vi "SpinnyCloseMotor.vi"(0 "Arduino Resource":T1={"VISA resource"="", "Board Type"=enum."Uno", "Connection Type"=enum."USB / Serial", "Bytes Per Packet (15)"=15}, 5 "error in":errorcluster) -> ()   [LabVIEW 2014]
uses:
  <vilib>/LabVIEW Interface for Arduino/Type Defs/Arduino Resource.ctl
  <vilib>/LabVIEW Interface for Arduino/Type Defs/Board Type.ctl
  <vilib>/LabVIEW Interface for Arduino/LabVIEW Interface for Arduino.lvlib
panel:
  in  "Stepper #":u8=1
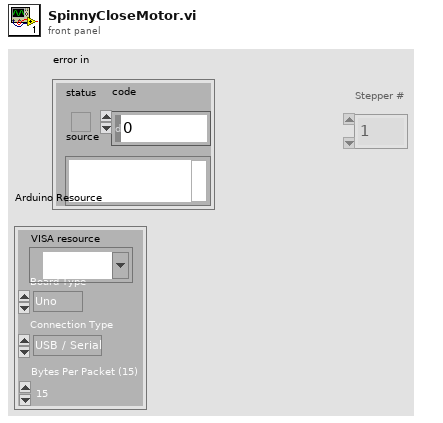
[diagram p1: front panel]
types:
  T1 = typedef "LabVIEW Interface for Arduino.lvlib/Arduino Resource.ctl" = cluster{"VISA resource":refnum<visa-resource-name>, "Board Type":T2, "Connection Type":enum8{"USB / Serial"}, "Bytes Per Packet (15)":u8}
  T2 = typedef "LabVIEW Interface for Arduino.lvlib/Board Type.ctl" = enum16{"Uno", "Dimuelanove w/Atmega 328", "Mega 2560"}
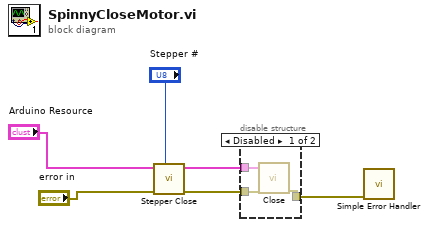
[diagram p0: block diagram]
diagram:
  n1 = call <vilib>:"Stepper Close.vi"("Stepper #"="Stepper #", "error in"="error in", "Arduino Resource"="Arduino Resource") -> ("error out"=w2:errorcluster, "Arduino Resource Out"=w3:T1)  [unwired: 7 in]
  n2 = disable-structure shown="Disabled" {
    disable-tunnel: w3 -> [w9 _]
    disable-tunnel: w2 -> [w8 _]
    disable-tunnel: [w7 _] -> w1
    frame Disabled {
      n3 = call <vilib>:"Close.vi"("Arduino Resource"=w9, "error in"=w8) -> ("error out"=w7:errorcluster)  [unwired: 13 in]
    }
    frame Enabled {
    }
  }
  n4 = call <vilib>:"Simple Error Handler.vi"("error in (no error)"=w1) -> ()  [unwired: 4 in, 5 out]
